vi "build tempo map.vi"(8 "error in (no error)":errorcluster, 11 "midi-file-events in":refnum<class "midi-file-events.lvclass">) -> (0 "error out":errorcluster, 3 "midi-file-events out":refnum<class "midi-file-events.lvclass">)   [LabVIEW 2020, in "midi-file-events.lvclass"]
uses:
  midi-file-events.lvclass
  midi-file-events.lvclass/midi-file-events.ctl
  midi-file-event/midi-file-event.lvclass/midi-file-event.ctl
  midi-file-event/Delta Tiime.get.vi
  midi-file-event/midi-file-event.lvclass
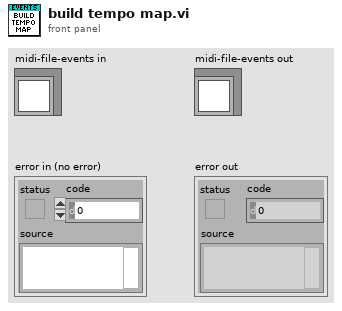
[diagram p1: front panel]
types:
  T1 = typedef "midi-file-events.lvclass/privatedata.ctl" = cluster{"ticks per quarter note (division)":i16, "Tempo Map":map{dbl, dbl}, "Track data by Track number":map{i32, map{dbl, set{refnum<class "midi-file-event.midi.lvclass">}}}}
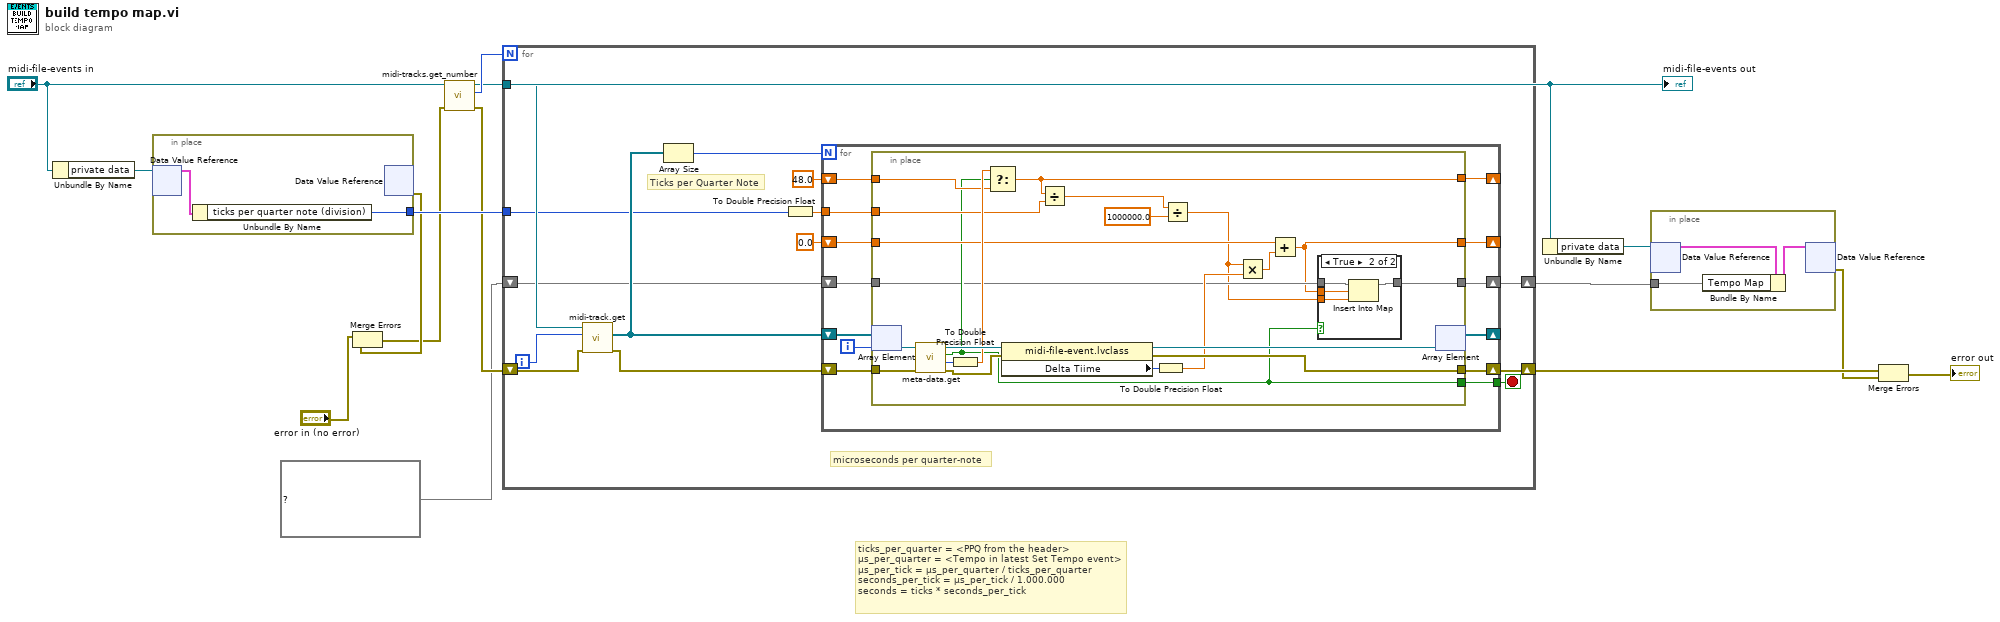
[diagram p0: block diagram]
diagram:
  # "ticks_per_quarter = <PPQ from the header>\nµs_per_quarter = <Tempo in latest Set Tempo event>\nµs_per_tick = µs_per_quarter / ticks_per_quarter\nseconds_per_tick = µs_per_tick / 1.000.000\nseconds = ticks * seconds_per_tick"
  n1 = Unbundle By Name("midi-file-events in") -> ("private data"=w14:refnum<data-value>)
  n2 = in-place {
    in-place-border: [w16] -> w13
    n3 = in-place-dvr #1(w14) -> (w17:T1)  [unwired: 1 out]
    n4 = Unbundle By Name(w17) -> ("ticks per quarter note (division)"=w16:i16)
    n5 = in-place-dvr #1() -> (w10:errorcluster)  [unwired: 1 in, 1 out]
  }
  n6 = Merge Errors("error in (no error)", w10) -> (w9:errorcluster)
  n7 = call "midi-tracks.get_number.vi"("error in (no error)"=w9, "midi-file-events in"="midi-file-events in") -> ("error out"=w8:errorcluster, "Numer of Tracks"=w15:i32, "midi-file-events out"=w5:refnum<class "midi-file-events.lvclass">)  [unwired: 7 in]
  "midi-file-events out" <- w5
  n8 = for {
    N: w15 -> [_]
    tunnel: w5 -> [w26]
    tunnel: w13 -> [w24]
    shift-right: [w20] -> w3
    shift-left: w8 -> [w22]
    shift-right: [w18] -> w4
    shift-left: map{dbl, dbl} {} ("map") -> [w19]
    i -> [w25]
    stop <- w23 stop-if-true
    # "microseconds per quarter-note"
    # "Ticks per Quarter Note"
    n9 = call "midi-track.get.vi"("error in (no error)"=w22, "Track Number"=w25, "midi-file-events in"=w26) -> ("error out"=w21:errorcluster, "file events"=w31:refnum<class "midi-file-event.lvclass">[])  [unwired: 6 in, 1 out]
    n10 = Array Size(array=w31) -> (size(s)=w30:i32)
    n11 = To Double Precision Float(number=w24) -> (double precision float=w28:dbl)
    n12 = for {
      N: w30 -> [_]
      shift-right: [w43] -> _
      shift-left: w31 -> [w44]
      tunnel: w28 -> [w42]
      shift-right: [w41] -> _
      shift-left: 48.0 ("microseconds per quarter note") -> [w40]
      shift-right: [w38] -> _
      shift-left: 0.0 ("microseconds per quarter note") -> [w39]
      tunnel: [w36] -> w23
      shift-right: [w34] -> w20
      shift-left: w21 -> [w35]
      shift-right: [w32] -> w18
      shift-left: w19 -> [w33]
      i -> [w37]
      n13 = in-place {
        in-place-border: w42 -> [w52]
        in-place-border: [w53] -> w41
        in-place-border: w40 -> [w57]
        in-place-border: w39 -> [w60]
        in-place-border: [w46] -> w38
        in-place-border: [w49] -> w36
        in-place-border: w35 -> [w56]
        in-place-border: [w54] -> w34
        in-place-border: w33 -> [w48]
        in-place-border: [w47] -> w32
        n14 = in-place-array #2(w44, w37) -> (w66:refnum<class "midi-file-event.lvclass">)
        n15 = call "meta-data.get.vi"("error in (no error)"=w56, "midi-file-event in"=w66) -> ("error out"=w55:errorcluster, "microseconds per quarter note"=w58:i32, "New Tempo"=w49:bool, "midi-file-event out"=w65:refnum<class "midi-file-event.lvclass">)  [unwired: 6 in]
        n16 = To Double Precision Float(number=w58) -> (double precision float=w63:dbl)
        n17 = Select(t=w63, s=w49, f=w57) -> (s? t:f=w53:dbl)
        n18 = property class="midi-file-event.lvclass"(reference=w65, error in=w55) -> (reference out=w61:refnum<class "midi-file-event.lvclass">, error out=w54:errorcluster, "Delta Tiime"=w62:u32)
        n19 = Divide(x=w53, y=w52) -> (x/y=w51:dbl)
        n20 = To Double Precision Float(number=w62) -> (double precision float=w50:dbl)
        n21 = Divide(x=w51, y=1000000.0) -> (x/y=w45:dbl)
        n22 = Multiply(x=w45, y=w50) -> (x*y=w59:dbl)
        n23 = Add(x=w60, y=w59) -> (x+y=w46:dbl)
        n24 = case shown="True" w49 {
          tunnel: w48 -> [w67 w71]
          tunnel: [w67 w70] -> w47
          tunnel: w46 -> [_ w69]
          tunnel: w45 -> [_ w68]
          frame False {
          }
          frame True {
            n25 = Insert Into Map(map in=w71, key=w69, value=w68) -> (map out=w70:map{dbl, dbl})  [unwired: 2 out]
          }
        }
        n26 = in-place-array #2(w61) -> (w43:refnum<class "midi-file-event.lvclass">[])  [unwired: 1 out]
      }
    }
  }
  n27 = Unbundle By Name(w5) -> ("private data"=w6:refnum<data-value>)
  n28 = in-place {
    in-place-border: w4 -> [w72]
    n29 = in-place-dvr #3(w6) -> (w74:T1)  [unwired: 1 out]
    n30 = Bundle By Name(cluster=w74, "Tempo Map"=w72) -> (w73:T1)
    n31 = in-place-dvr #3(w73) -> (w2:errorcluster)  [unwired: 1 out]
  }
  n32 = Merge Errors(w3, w2) -> (→"error out":errorcluster)
